vi "serialization tests.vi"() -> ()   [LabVIEW 2013, in "scan engine tests.lvlib"]
uses:
  scan engine tests.lvlib
  configuration/Scan Engine configuration.lvclass
panel:
  out "rates equal":bool
  out "channels equal":bool
  out "no error":errorcluster
  out "no error":errorcluster
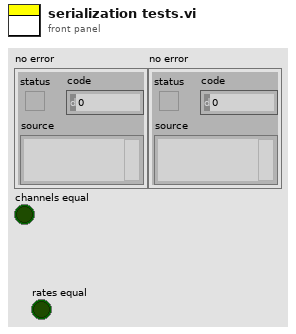
[diagram p1: front panel]
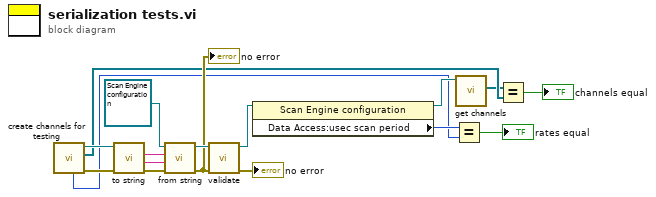
[diagram p0: block diagram]
diagram:
  n1 = call "create channels for testing.vi"() -> ("error out"=w5:errorcluster, "chans"=w3:refnum<class "TBM channel.lvclass">[], "Scan Engine configuration out"=w6:refnum<class "Scan Engine configuration.lvclass">, "usec scan period"=w1:u32)  [unwired: 7 in, 1 out]
  n2 = call-dynamic "to string.vi"("error in"=w5, "Scan Engine configuration in"=w6) -> ("error out"=w17:errorcluster, "data"=w16:string, "version"=w15:string)  [unwired: 6 in, 1 out]
  n3 = call-dynamic "from string.vi"("error in"=w17, "data"=w16, "version"=w15, "Scan Engine configuration in"=refnum<class "Scan Engine configuration.lvclass"> refnum ("Scan Engine configuration")) -> ("error out"=w12:errorcluster, "Scan Engine configuration out"=w14:refnum<class "Scan Engine configuration.lvclass">)  [unwired: 6 in]
  "no error" <- w12
  n4 = call-dynamic "validate.vi"("error in"=w12, "Scan Engine configuration in"=w14) -> ("error out"=→"no error":errorcluster, "Scan Engine configuration out"=w10:refnum<class "Scan Engine configuration.lvclass">)  [unwired: 8 in]
  n5 = property class="Scan Engine configuration"(reference=w10) -> (reference out=w4:refnum<class "Scan Engine configuration.lvclass">, "Data Access:usec scan period"=w8:u32)  [unwired: 1 in, 1 out]
  n6 = Equal?(x=w8, y=w1) -> (x = y?=→"rates equal":bool)
  n7 = call-dynamic "get channels.vi"("module configuration in"=w4) -> ("channels"=w2:refnum<class "TBM channel.lvclass">[])  [unwired: 9 in, 1 out]
  n8 = Equal?(x=w2, y=w3) -> (x = y?=→"channels equal":bool)
